vi "Display.vi"(8 "error in":errorcluster, 11 "Timeout in":refnum<class "Timeout.lvclass">) -> (0 "error out":errorcluster, 3 "Timeout out":refnum<class "Timeout.lvclass">)   [LabVIEW 2021, in "Pop-Up.lvlib" / "Timeout.lvclass"]
doc: "This vi displays the timeout Popup.\n\n<b>Code Developed By:</b> +\nDaniel Coons +\nhttps://github.com/danielcoons/tsc-pop-up"
uses:
  Timeout.lvclass
  C:/Development/Open Source/tsc-pop-up/Popup/Popup.lvclass
  Timeout.lvclass/Timeout.ctl
  Popup/Popup.lvclass/Popup.ctl
  Popup/Data Member Access/Read Theme.vi
  Theme/Theme.lvclass
  Popup/Popup.lvclass
  user32.dll
panel:
  out "header":bool
  out "count":string
  out "2D Picture":picture
  out "String":string
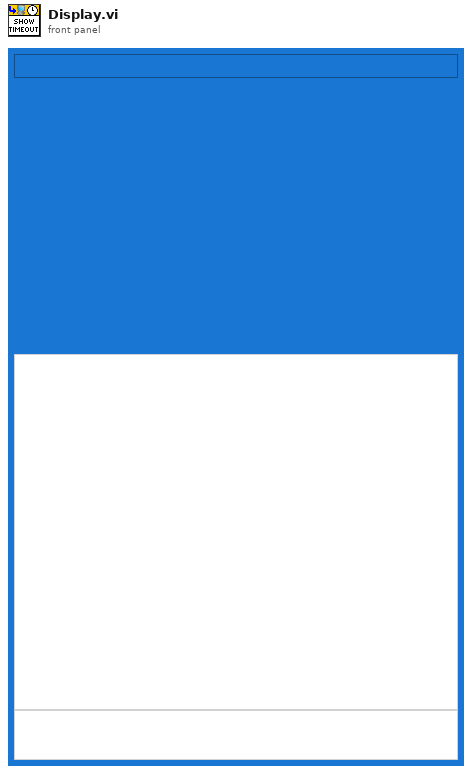
[diagram p1: front panel]
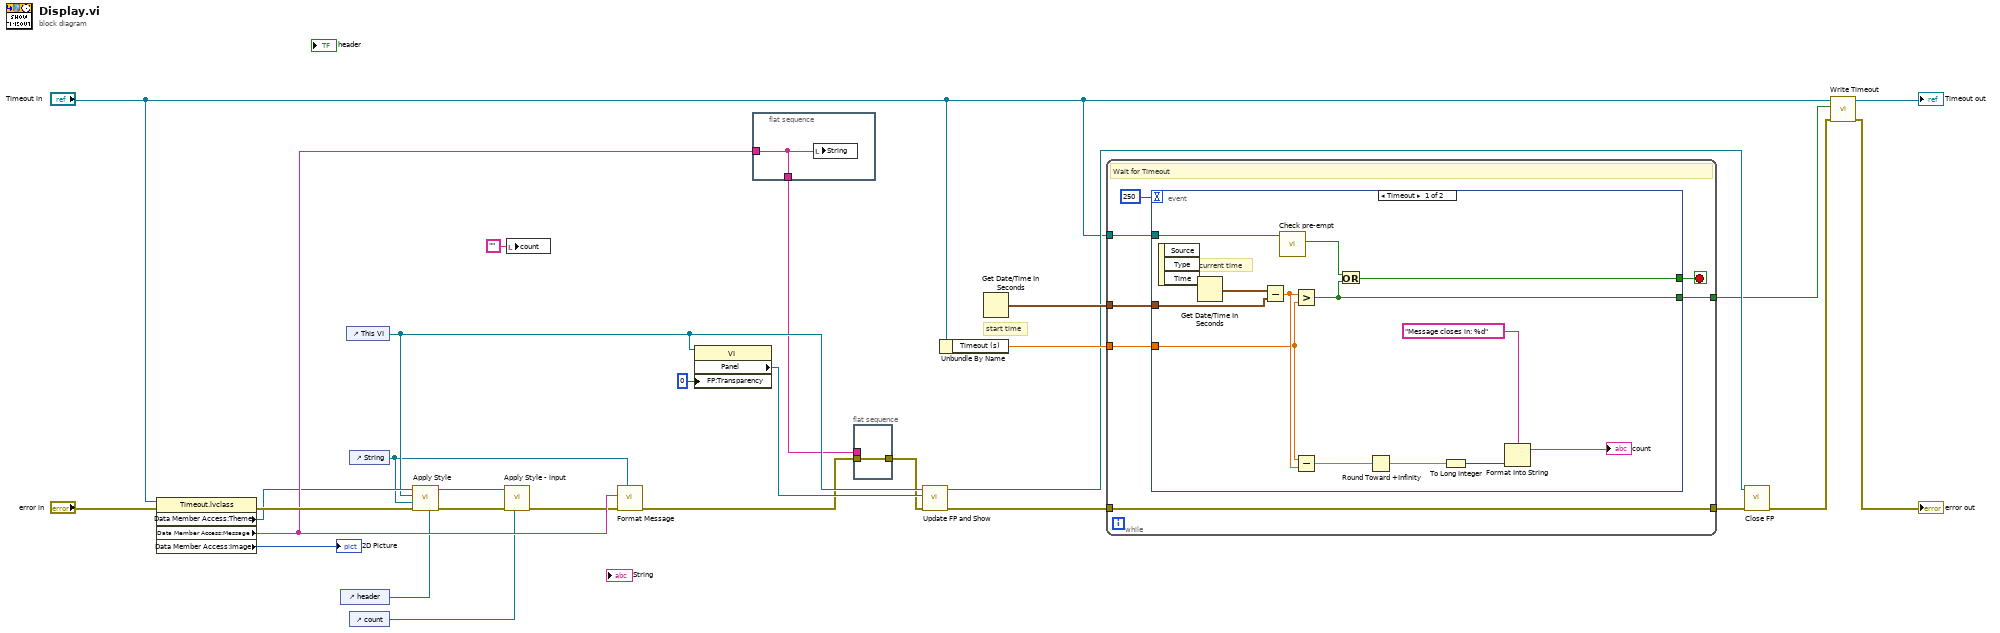
[diagram p0: block diagram]
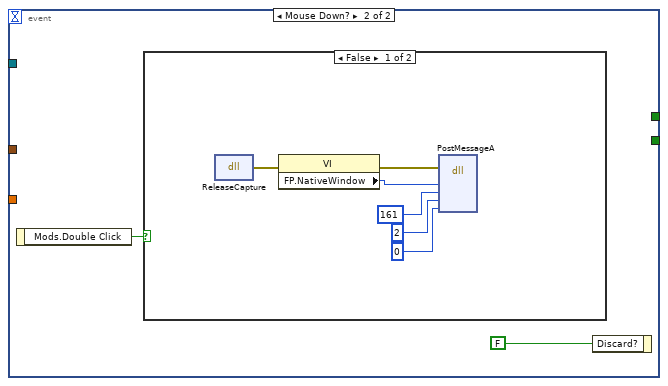
[diagram p2: hidden frame]
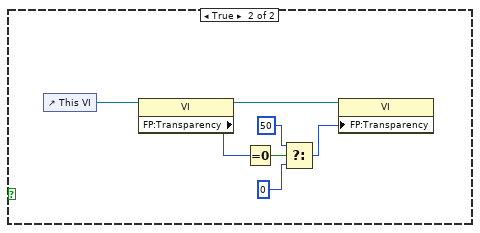
[diagram p3: hidden frame]
diagram:
  # "start time"
  n1 = property class="Timeout.lvclass"(reference="Timeout in", error in="error in") -> (error out=w25:errorcluster, "Data Member Access:Theme"=w16:refnum<class "Theme.lvclass">, "Data Member Access:Message"=w18:string, "Data Member Access:Image"=→"2D Picture":picture)  [unwired: 1 out]
  n2 = control-ref of="header"() -> (w13:refnum<vi>)
  n3 = control-ref of="This VI"() -> (w15:refnum<vi>)
  n4 = control-ref of="String"() -> (w14:refnum<vi>)
  n5 = control-ref of="count"() -> (w10:refnum<vi>)
  n6 = call "Apply Style.vi"("header ref"=w13, "error in"=w25, "message ref"=w14, "pop up ref"=w15, "Theme in"=w16) -> ("error out"=w17:errorcluster, "Theme out"=w11:refnum<class "Theme.lvclass">)  [unwired: 5 in]
  n7 = call "Apply Style - input.vi"("input ref"=w10, "error in (no error)"=w17, "Theme in"=w11) -> ("error out"=w12:errorcluster)  [unwired: 7 in, 1 out]
  n8 = local write "count"("" ("count")) -> ()
  n9 = call "Format Message.vi"("formatted string"=w14, "error in"=w12, "String Input"=w18) -> ("error out"=w3:errorcluster)  [unwired: 7 in, 1 out]
  n10 = property class="VI"(reference=w15, "FP:Transparency"=u8 0 ("Front Panel Window:Transparency")) -> ("Panel"=w21:refnum<vi>)  [unwired: 1 in, 2 out]
  n11 = flat-sequence {
    tunnel: [w29] -> w1
    tunnel: w18 -> [w29]
    frame #0 {
      n12 = local write "String"(w29) -> ()
    }
  }
  n13 = flat-sequence {
    tunnel: w3 -> [w30]
    tunnel: [w30] -> w2
    tunnel: w1 -> [_]
    frame #0 {
    }
  }
  n14 = call "Update FP and Show.vi"("error in (no error)"=w2, "Panel Ref"=w21, "VI in"=w15) -> ("error out"=w22:errorcluster, "VI out"=w20:refnum<vi>)  [unwired: 7 in]
  n15 = Unbundle By Name("Timeout in") -> ("Timeout (s)"=w26:dbl)
  n16 = Get Date/Time In Seconds() -> (seconds since 1Jan1904=w27:timestamp)
  n17 = while {
    tunnel: [w33] -> w28
    tunnel: w22 -> [w33]
    tunnel: w27 -> [w37]
    tunnel: w26 -> [w36]
    tunnel: "Timeout in" -> [w34]
    tunnel: [w31] -> w4
    stop <- w35 stop-if-true
    # "Wait for Timeout"
    n18 = event shown="[0] Timeout" {
      selector: _ -> [_ _]
      dyn-events: _ -> [_ _]
      timeout: 250 -> [_ _]
      tunnel: w37 -> [w50 _]
      tunnel: w36 -> [w47 _]
      tunnel: [w44 _] -> w35
      tunnel: w34 -> [w42 _]
      tunnel: [w38 _] -> w31
      event Timeout {
        # "current time"
        n19 = event-data() -> ()  [unwired: 1 in, 3 out]
        n20 = Get Date/Time In Seconds() -> (seconds since 1Jan1904=w49:timestamp)
        n21 = Subtract(x=w49, y=w50) -> (x-y=w48:dbl)
        n22 = call "Check pre-empt.vi"("_Popup in"=w42) -> ("Pre-empted?"=w43:bool)  [unwired: 8 in, 2 out]
        n23 = Greater?(x=w48, y=w47) -> (0:w38:bool)
        n24 = Subtract(x=w47, y=w48) -> (x-y=w45:dbl)
        n25 = Or(x=w43, y=w38) -> (x .or. y?=w44:bool)
        n26 = Round Toward +Infinity(x=w45) -> (ceil(x): smallest int >= x=w40:dbl)
        n27 = To Long Integer(number=w40) -> (32bit integer=w41:i32)
        n28 = Format Into String(format string="Message closes in: %d", w41) -> (resulting string=→"count":string)  [unwired: 2 in, 1 out]
      }
      event Mouse Down? {
        n29 = event-data() -> ("Mods.Double Click"=w51:bool)  [unwired: 1 in]
        n30 = case shown="False" w51 {
          frame False {
            n31 = dll-call lib="user32.dll" fn="ReleaseCapture"() -> (error out=w56:errorcluster)  [unwired: 4 in, 1 out]
            n32 = property class="VI"(error in=w56) -> (error out=w57:errorcluster, "FP.NativeWindow"=w58:u64)  [unwired: 1 in, 1 out]
            n33 = dll-call lib="user32.dll" fn="PostMessageA"(error in=w57, "hWnd"=w58, "Msg"=161, "wParam"=2, "lParam"=0) -> ()  [unwired: 7 in, 2 out]
          }
          frame True {
            n34 = control-ref of="This VI"() -> (w65:refnum<vi>)
            n35 = property class="VI"(reference=w65) -> (reference out=w63:refnum<vi>, "FP:Transparency"=w64:u8)  [unwired: 1 in, 1 out]
            n36 = Equal To 0?(x=w64) -> (x = 0?=w62:bool)
            n37 = Select(t=u8 50, s=w62, f=u8 0) -> (s? t:f=w59:u8)
            n38 = property class="VI"(reference=w63, "FP:Transparency"=w59) -> ()  [unwired: 1 in, 2 out]
          }
        }
        n39 = event-data("Discard?"=FALSE) -> ()  [unwired: 1 in, 1 out]
      }
    }
  }
  n40 = call "Close FP.vi"("error in (no error)"=w28, "VI in"=w20) -> ("error out"=w6:errorcluster)  [unwired: 9 in]
  n41 = call "Write Timeout.vi"("error in"=w6, "Timeout?"=w4, "Popup in"="Timeout in") -> ("error out"=→"error out":errorcluster, "Popup out"=→"Timeout out":refnum<class "Timeout.lvclass">)  [unwired: 7 in]
